vi "Refresh Get ECU Name.vi"(8 "Type (Input)":T3, 9 "ECUs":T4[](array[typedef]), 10 "Refresh Frame":T1, 11 "Frames":T1[](array[typedef])) -> (3 "ECU Name":string)   [LabVIEW 2020, in "Communication Bus Template System Explorer.lvlib" / "Implementation.lvlib"]
uses:
  Implementation.lvlib
  Types/ECU.ctl
  <vilib>/NI VeriStand/Custom Device API/Custom Device Channel Type.ctl
  Types/Refresh Frame.ctl
  Types/Refresh Signal.ctl
  <vilib>/NI VeriStand/Custom Device API/Custom Device API.lvlib
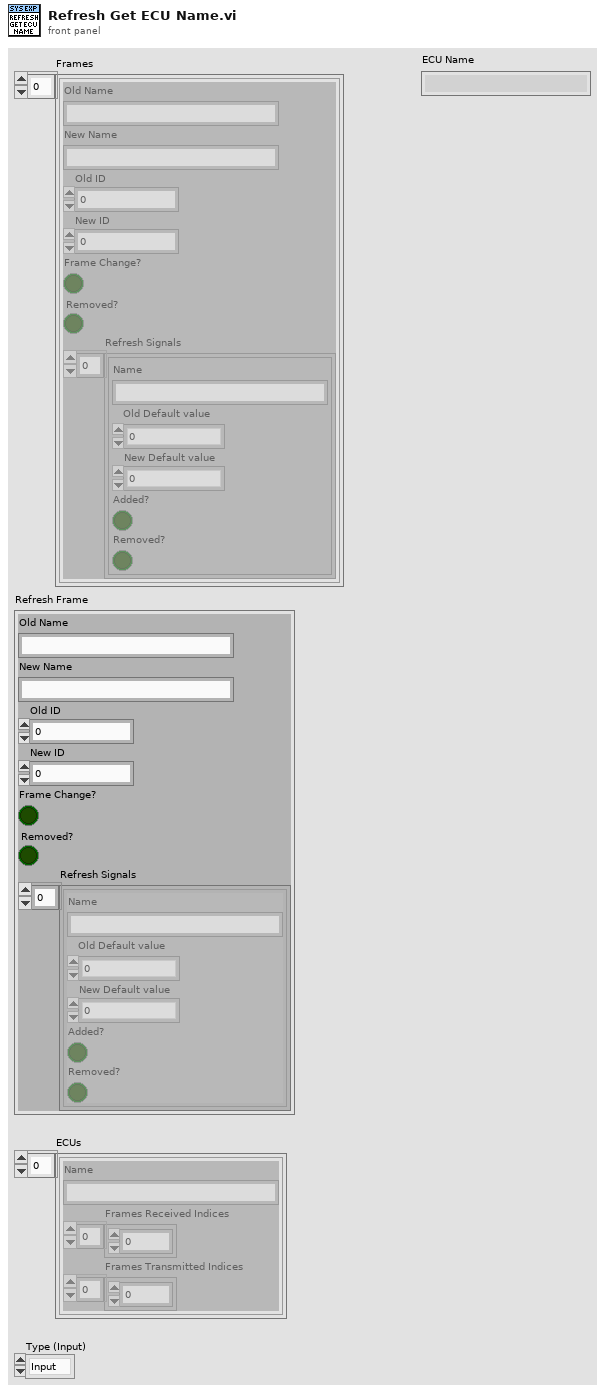
[diagram p1: front panel]
types:
  T1 = typedef "Communication Bus Template System Explorer.lvlib/Implementation.lvlib/Refresh Frame.ctl" = cluster{"Old Name":string, "New Name":string, "Old ID":u32, "New ID":u32, "Frame Change?":bool, "Removed?":bool, "Refresh Signals":T2[]}
  T2 = typedef "Communication Bus Template System Explorer.lvlib/Implementation.lvlib/Refresh Signal.ctl" = cluster{"Name":string, "Old Default value":dbl, "New Default value":dbl, "Added?":bool, "Removed?":bool}
  T3 = typedef "Custom Device API.lvlib/Custom Device Channel Type.ctl" = enum16{"Input", "Output"}
  T4 = typedef "Communication Bus Template System Explorer.lvlib/Implementation.lvlib/ECU.ctl" = cluster{"Name":string, "Frames Received Indices":u32[], "Frames Transmitted Indices":u32[]}
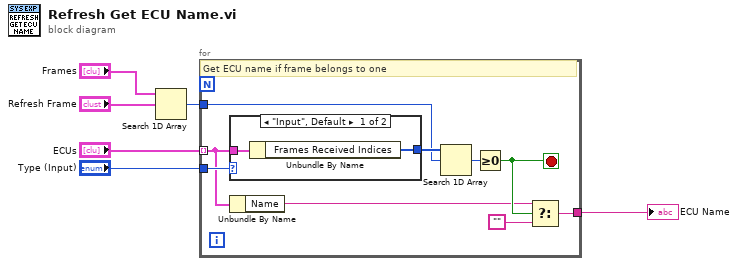
[diagram p0: block diagram]
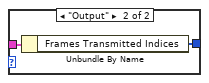
[diagram p2: hidden frame]
diagram:
  n1 = Search 1D Array(1D array="Frames", element="Refresh Frame") -> (index of element=w6:i32)  [unwired: 1 in]
  n2 = for {
    tunnel: w6 -> [w12]
    tunnel: "ECUs" -> [w14] mode=indexing
    tunnel: "Type (Input)" -> [w15]
    tunnel: [w7] -> w1
    stop <- w10 stop-if-true
    # "Get ECU name if frame belongs to one"
    n3 = case shown="\"Input\", Default" w15 {
      tunnel: w14 -> [w17 w19]
      tunnel: [w16 w18] -> w13
      frame "Input", Default {
        n4 = Unbundle By Name(w17) -> ("Frames Received Indices"=w16:u32[])
      }
      frame "Output" {
        n5 = Unbundle By Name(w19) -> ("Frames Transmitted Indices"=w18:u32[])
      }
    }
    n6 = Unbundle By Name(w14) -> ("Name"=w9:string)
    n7 = Search 1D Array(1D array=w13, element=w12) -> (index of element=w11:i32)  [unwired: 1 in]
    n8 = Greater Or Equal To 0?(x=w11) -> (x >= 0?=w10:bool)
    n9 = Select(t=w9, s=w10, f="") -> (s? t:f=w7:string)
  }
  "ECU Name" <- w1
